vi "PH_BlackBox.panel.vi"(0 "object ref":refnum<vi>, 5 "error in (no error)":errorcluster) -> (19 "error out":errorcluster)   [LabVIEW 2014, in "PH_BlackBox.lvlib"]
doc: "By this VI a ross relais can be monitored and switched. \n\nThe indicators \"CLOSED\", \"OPEN\" and \"SWITCH STATE\" show the value of the Beckhoff-Tag: blue indicates bad tag status reference problems, darkgreen false and lightgreen on. If everything is working fine, \"CLOSED\" and \"SWITCH STATE\" should show the same value, while \"OPEN\" has the opposite value. \n\nThe oval button switches the ross relais. It should be in the same state as the \"SWITCH STATE\" indicator. \n\n\"EXIT\" closes the front panel (GUI), while \"Delete Instance\" disconnects and removes the instance from the PCS.\n\nThis VI has no machine safety relevant logig: there is neither a check of internal conclict nor with other objects, for example conflict with other ross relais. Therefore it must be handled with care and should be operated by well educated operators only. It is forseen exclusively for direct operating and testing of the system. \n\nLicense Agreement for this software:\n\nCopyright (C)\nGesellschaft für Schwerionenforschung, GSI\nPlanckstr. 1\n64291 Darmstadt\nGermany\n\nContact: D.Beck@gsi.de \n\nThis program is free software; you can redistribute it and/or modify it under the terms of the GNU General Public License as published by the Free Software Foundation; either version 2 of the license, or (at your option) any later version.\n\nThis program is distributed in the hope that it will be useful, but WITHOUT ANYW ARRANTY; without even the implied warranty of MERCHANTABILITY or FITNESS FOR A PARTICULAR PURPOSE. See the GNU General License for more details (http://www.gnu.org).\n\nGesellschaft für Schwerionenforschung, GSI\nPlanckstr. 1, 64291 Darmstadt, Germany\nFor all questions and ideas contact: M.Richter@gsi.de, H.Brand@gsi.de or D.Beck@gsi.de.\nLast update: 18-DEC-2002"
uses:
  PH_BlackBox.lvlib
  PH_StatusHandler/PH_StatusHandler.GUI element.ctl
  PH_BlackBox.GUI Refs.ctl
  CSCore/CSObj/CSObj.lvlib
  CSCore/CSSystem/CSSystemLib/CSSystemLib.lvlib
  PH_Common/PH_Common.lvlib
  PH_PSDBWriter/PH_PSDBWriter.lvlib
  PH_Class/PH_Class.lvlib
  PH_StatusHandler/PH_StatusHandler.lvlib
panel:
  out "Textfield":string="Testtext"
  out "PSDB Status":u32(colorbox)=6618880 caption="PSDB"
  out "Status":T1 caption="Enabling State"
  out "POWER ON":u32(colorbox)
  in  "Move in":bool caption="Dir"
  in  "Move":bool
  out "REMOTE":u32(colorbox)
  out "OUT":u32(colorbox)
  in  "Delete":bool
  out "IN":u32(colorbox)
  out "MOVE":u32(colorbox)
  out "MOVE IN":u32(colorbox)
  in  "Exit":bool
  out "loop counter":i32
  # "PCS"
  # "3.40"
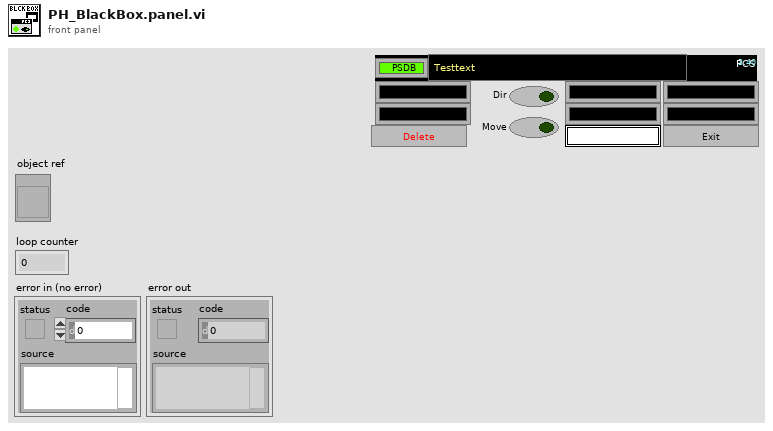
[diagram p1: front panel]
types:
  T1 = typedef "PH_StatusHandler.lvlib/PH_StatusHandler.GUI element.ctl" = u16
  T2 = typedef "PH_BlackBox.lvlib/PH_BlackBox.GUI Refs.ctl" = cluster{"MOVE IN":refnum<vi>, "MOVE":refnum<vi>, "IN":refnum<vi>, "OUT":refnum<vi>, "REMOTE":refnum<vi>, "GUI-Knob Move":refnum<vi>, "GUI-Knob Move in":refnum<vi>, "POWER ON":refnum<vi>, "Delete":refnum<vi>, "Function Textfield":refnum<vi>}
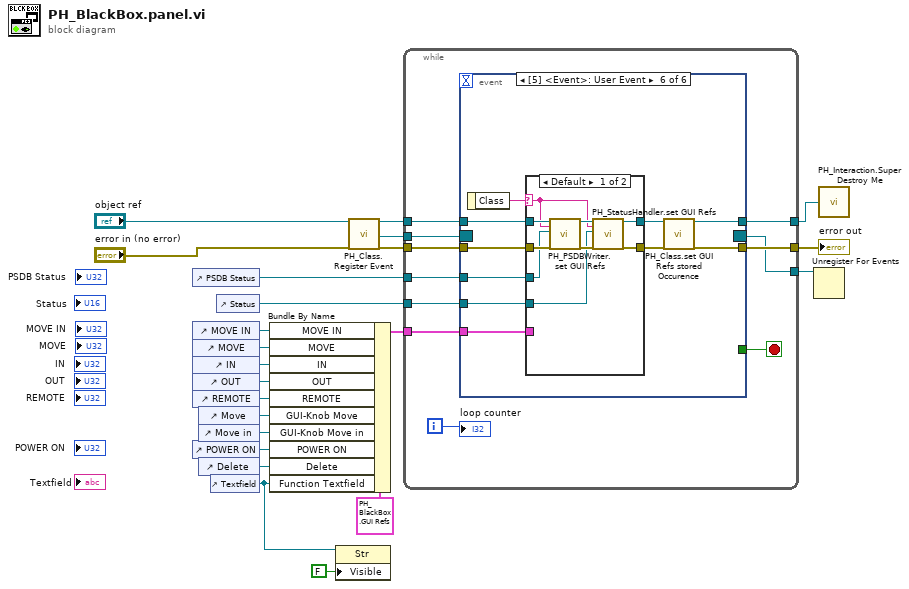
[diagram p0: block diagram]
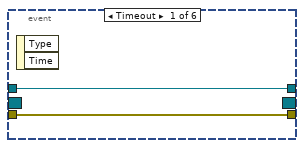
[diagram p2: hidden frame]
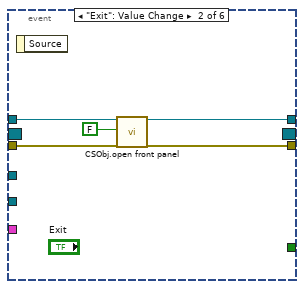
[diagram p3: hidden frame]
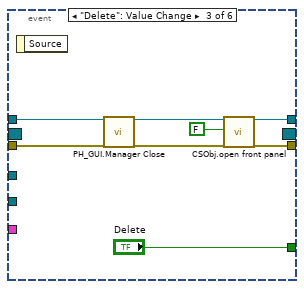
[diagram p4: hidden frame]
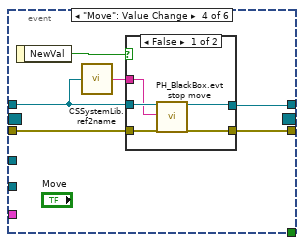
[diagram p5: hidden frame]
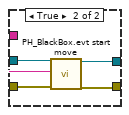
[diagram p6: hidden frame]
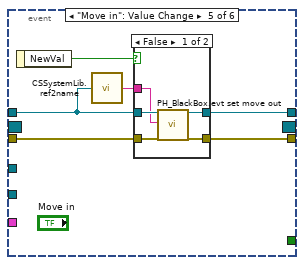
[diagram p7: hidden frame]
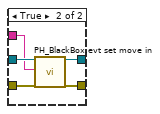
[diagram p8: hidden frame]
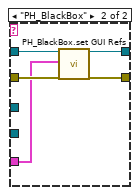
[diagram p9: hidden frame]
diagram:
  n1 = control-ref of="PSDB Status"() -> (w9:refnum<vi>)
  n2 = control-ref of="MOVE IN"() -> (w23:refnum<vi>)
  n3 = control-ref of="MOVE"() -> (w22:refnum<vi>)
  n4 = control-ref of="IN"() -> (w21:refnum<vi>)
  n5 = control-ref of="OUT"() -> (w20:refnum<vi>)
  n6 = control-ref of="REMOTE"() -> (w17:refnum<vi>)
  n7 = control-ref of="POWER ON"() -> (w16:refnum<vi>)
  n8 = control-ref of="Move"() -> (w19:refnum<vi>)
  n9 = control-ref of="Move in"() -> (w18:refnum<vi>)
  n10 = control-ref of="Delete"() -> (w15:refnum<vi>)
  n11 = control-ref of="Textfield"() -> (w3:refnum<vi>)
  n12 = control-ref of="Status"() -> (w1:refnum<vi>)
  n13 = Bundle By Name(cluster=T2 {"MOVE IN"=refnum, "MOVE"=refnum, "IN"=refnum, "OUT"=refnum, "REMOTE"=refnum, "GUI-Knob Move"=refnum, "GUI-Knob Move in"=refnum, "POWER ON"=refnum, "Delete"=refnum, "Function Textfield"=refnum} ("GUI Refs"), "MOVE IN"=w23, "MOVE"=w22, "IN"=w21, "OUT"=w20, "REMOTE"=w17, "GUI-Knob Move"=w19, "GUI-Knob Move in"=w18, "POWER ON"=w16, "Delete"=w15, "Function Textfield"=w3) -> (w4:T2)
  n14 = property class="Str"(reference=w3, "Visible"=FALSE) -> ()  [unwired: 1 in, 2 out]
  n15 = call "PH_Class.Register Event.vi"("i ref in"="object ref", "error in (no error)"="error in (no error)") -> ("i ref out"=w12:refnum<vi>, "Event Registration Refnum"=w10:refnum<event-registration>, "error out"=w11:errorcluster)  [unwired: 15 in]
  n16 = while {
    tunnel: w12 -> [w30]
    tunnel: [w29] -> w14
    tunnel: w11 -> [w32]
    tunnel: [w31] -> w13
    tunnel: w10 -> [w26]
    tunnel: w9 -> [w28]
    tunnel: [w25] -> w8
    tunnel: w4 -> [w27]
    tunnel: w1 -> [w24]
    i -> [w33]
    stop <- w34 stop-if-true
    n17 = event shown="[5] <Event>: User Event" {
      selector: w26 -> [_ _ _ _ _ _]
      dyn-events: [_ _ _ _ _ _] -> w25
      timeout: _ -> [_ _ _ _ _ _]
      tunnel: [_ _ "Delete" _ _ _] -> w34
      tunnel: w30 -> [w35 w41 w43 w53 w69 w91]
      tunnel: w32 -> [w36 w39 w45 w54 w71 w90]
      tunnel: [w36 w38 w47 w51 w70 w85] -> w31
      tunnel: [w35 w37 w46 w50 w68 w83] -> w29
      tunnel: w28 -> [_ _ _ _ _ w87]
      tunnel: w27 -> [_ _ _ _ _ w86]
      tunnel: w24 -> [_ _ _ _ _ w82]
      event Timeout {
        n18 = event-data() -> ()  [unwired: 1 in, 2 out]
      }
      event "Exit": Value Change {
        n19 = event-data() -> ()  [unwired: 1 in, 1 out]
        n20 = call "CSObj.open front panel.vi"("i ref in"=w41, "frontPanelOpen"=FALSE ("front panel open"), "error in (no error)"=w39) -> ("i ref out"=w37:refnum<vi>, "error out"=w38:errorcluster)  [unwired: 15 in]
      }
      event "Delete": Value Change {
        n21 = event-data() -> ()  [unwired: 1 in, 1 out]
        n22 = call "PH_GUI.Manager Close.vi"("i ref in"=w43, "error in"=w45) -> ("i ref out"=w42:refnum<vi>, "error out"=w44:errorcluster)  [unwired: 16 in]
        n23 = call "CSObj.open front panel.vi"("i ref in"=w42, "frontPanelOpen"=FALSE ("front panel open"), "error in (no error)"=w44) -> ("i ref out"=w46:refnum<vi>, "error out"=w47:errorcluster)  [unwired: 15 in]
      }
      event "Move": Value Change {
        n24 = event-data() -> ("NewVal"=w55:bool)  [unwired: 1 in]
        n25 = call "CSSystemLib.ref2name.vi"("obj refnum"=w53) -> ("name"=w52:string)
        n26 = case shown="False" w55 {
          tunnel: w53 -> [w60 w65]
          tunnel: w54 -> [w59 w64]
          tunnel: w52 -> [w58 w62]
          tunnel: [w57 w63] -> w51
          tunnel: [w56 w61] -> w50
          frame False {
            n27 = call "PH_BlackBox.evt stop move.vi"("i ref in"=w60, "Instance"=w58, "error in (no error)"=w59) -> ("i ref out"=w56:refnum<vi>, "error out"=w57:errorcluster)  [unwired: 15 in]
          }
          frame True {
            n28 = call "PH_BlackBox.evt start move.vi"("i ref in"=w65, "Instance"=w62, "error in (no error)"=w64) -> ("i ref out"=w61:refnum<vi>, "error out"=w63:errorcluster)  [unwired: 15 in]
          }
        }
      }
      event "Move in": Value Change {
        n29 = event-data() -> ("NewVal"=w67:bool)  [unwired: 1 in]
        n30 = call "CSSystemLib.ref2name.vi"("obj refnum"=w69) -> ("name"=w66:string)
        n31 = case shown="False" w67 {
          tunnel: w69 -> [w76 w81]
          tunnel: w71 -> [w75 w80]
          tunnel: [w74 w79] -> w70
          tunnel: w66 -> [w73 w78]
          tunnel: [w72 w77] -> w68
          frame False {
            n32 = call "PH_BlackBox.evt set move out.vi"("i ref in"=w76, "Instance"=w73, "error in (no error)"=w75) -> ("i ref out"=w72:refnum<vi>, "error out"=w74:errorcluster)  [unwired: 15 in]
          }
          frame True {
            n33 = call "PH_BlackBox.evt set move in.vi"("i ref in"=w81, "Instance"=w78, "error in (no error)"=w80) -> ("i ref out"=w77:refnum<vi>, "error out"=w79:errorcluster)  [unwired: 15 in]
          }
        }
      }
      event User Event {
        n34 = event-data() -> ("Class"=w88:string)  [unwired: 1 in]
        n35 = case shown="Default" w88 {
          selector: w88 -> [w93 _]
          tunnel: w91 -> [w100 w105]
          tunnel: [w94 w103] -> w84
          tunnel: w90 -> [w99 w104]
          tunnel: [w96 w102] -> w89
          tunnel: w87 -> [w97 _]
          tunnel: w86 -> [_ w101]
          tunnel: w82 -> [w92 _]
          frame Default {
            n36 = call "PH_PSDBWriter.set GUI Refs.vi"("i ref in"=w100, "Class"=w93, "Ref PSDB Status"=w97, "error in"=w99) -> ("i ref out"=w95:refnum<vi>, "error out"=w98:errorcluster)  [unwired: 14 in]
            n37 = call "PH_StatusHandler.set GUI Refs.vi"("i ref in"=w95, "Class"=w93, "GUI Ref"=w92, "error in (no error)"=w98) -> ("i ref out"=w94:refnum<vi>, "error out"=w96:errorcluster)  [unwired: 14 in]
          }
          frame "PH_BlackBox" {
            n38 = call "PH_BlackBox.set GUI Refs.vi"("VI in"=w105, "GUI Refs"=w101, "error in (no error)"=w104) -> ("VI out"=w103:refnum<vi>, "error out"=w102:errorcluster)  [unwired: 15 in]
          }
        }
        n39 = call "PH_Class.set GUI Refs stored Occurence.vi"("i ref in"=w84, "error in (no error)"=w89) -> ("i ref out"=w83:refnum<vi>, "error out"=w85:errorcluster)  [unwired: 16 in]
      }
    }
    "loop counter" <- w33
  }
  "error out" <- w13
  n40 = Unregister For Events(event registration refnum=w8) -> ()  [unwired: 1 in, 1 out]
  n41 = call "PH_Interaction.Super Destroy Me.vi"("i ref out"=w14) -> ()
